vi "VelocityControl.vi"(10 "Power from PID":dbl format="%#_13g", 11 "Error":dbl format="%#_13g") -> (3 "Final Output":dbl)   [LabVIEW 2014]
uses:
  Typedefs/StackerStates.ctl
panel:
  in  "Stacker States":T1
  out "Power Output Cap":dbl
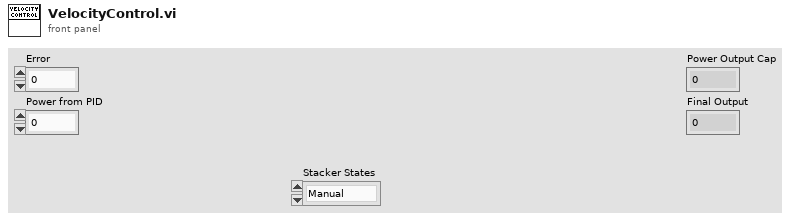
[diagram p1: front panel]
types:
  T1 = typedef "StackerStates.ctl" = enum16{"Manual ", "Hold", "Hold5", "Hold6", "GetTote", "DropStack", "Hover", "Hover5", "Wait for Up", "DecideHold", "DownTimerPeriod", "Prep Intake for Drop", "Check Arm before 5", "Make Arm ready for 5", "Check Arm before 6", "Make Arm ready for 6", "Delay for 5", "Delay for 6"}
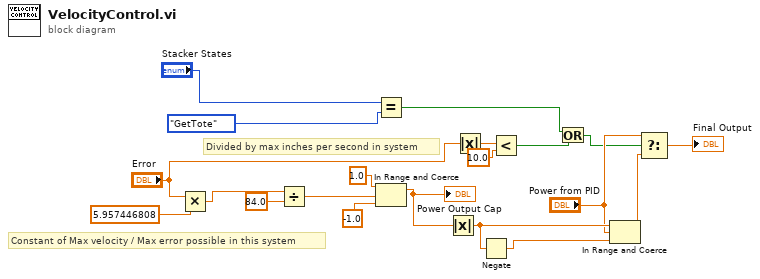
[diagram p0: block diagram]
diagram:
  # "Divided by max inches per second in system"
  # "Constant of Max velocity / Max error possible in this system"
  n1 = Multiply(x="Error", y=5.957446808) -> (x*y=w19:dbl)
  n2 = Divide(x=w19, y=84.0) -> (x/y=w13:dbl)
  n3 = Equal?(x="Stacker States", y=StackerStates."GetTote" ("Stacker States 2")) -> (x = y?=w2:bool)
  n4 = In Range and Coerce(upper limit=1.0, x=w13, lower limit=-1.0) -> (coerced(x)=w12:dbl)  [unwired: 1 out]
  "Power Output Cap" <- w12
  n5 = Absolute Value(x=w12) -> (abs(x)=w16:dbl)
  n6 = Absolute Value(x="Error") -> (abs(x)=w5:dbl)
  n7 = Negate(x=w16) -> (-x=w17:dbl)
  n8 = Less?(x=w5, y=10.0) -> (x < y?=w3:bool)
  n9 = Or(x=w2, y=w3) -> (x .or. y?=w1:bool)
  n10 = In Range and Coerce(upper limit=w16, x="Power from PID", lower limit=w17) -> (coerced(x)=w8:dbl)  [unwired: 1 out]
  n11 = Select(t="Power from PID", s=w1, f=w8) -> (s? t:f=→"Final Output":dbl)
